vi "Get Logging Interface.vi"(11 "Plugin Thread in":refnum<class "Plugin Thread.lvclass">) -> (2 "Logging Interface":refnum<class "Logging Interface.lvclass">, 3 "Plugin Thread out":refnum<class "Plugin Thread.lvclass">)   [LabVIEW 2019, in "DSF Core.lvlib" / "Plugin Thread.lvclass"]
uses:
  Thread/Plugin/Plugin Thread.lvclass
  Interface/Logging/Logging Interface.lvclass
  Thread/Plugin/Plugin Thread.lvclass/Plugin Thread.ctl
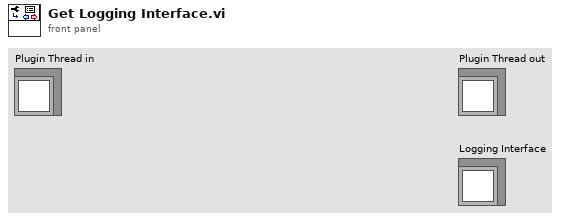
[diagram p1: front panel]
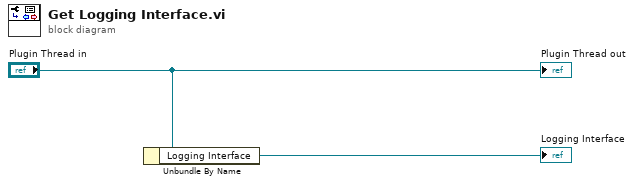
[diagram p0: block diagram]
diagram:
  n1 = Unbundle By Name("Plugin Thread in") -> ("Logging Interface"=→"Logging Interface":refnum<class "Logging Interface.lvclass">)
  "Plugin Thread out" <- "Plugin Thread in"
